vi "Build Version XML Prop Name.vi"(0 "NIPKG in":refnum<class "NIPKG_LV.lvclass">, 11 "error in (no error)":errorcluster) -> (4 "NIPKG out":refnum<class "NIPKG_LV.lvclass">, 6 "Version Number XML Prop Name":string, 15 "error out":errorcluster)   [LabVIEW 2017, in "CL_G3_VIComponentBuilder.lvlib" / "NIPKG_LV.lvclass"]
doc: "Returns the Version Number XML Property node name for an NI Package."
uses:
  NIPKG_LV.lvclass
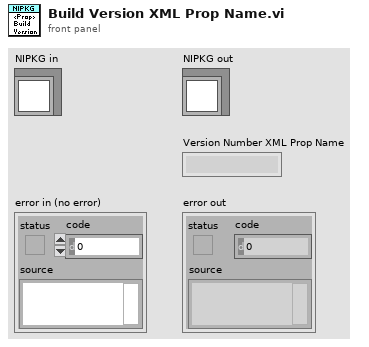
[diagram p1: front panel]
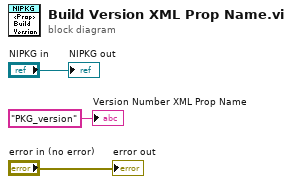
[diagram p0: block diagram]
diagram:
  "error out" <- "error in (no error)"
  "NIPKG out" <- "NIPKG in"
  "Version Number XML Prop Name" <- "PKG_version" ("Version Number XML Prop Name")
